vi "Format.vi"(5 "Force safe mode (false)":bool=TRUE caption="Force safe mode (true)", 7 "Restart after format (true)":bool caption="Restart after format (false)", 8 "error in (no error)":errorcluster, 10 "Network settings (reset all adapters)":T1=2 caption="Network settings (preserve all network adapters)" items=["reset primary, disable others", "preserve primary, disable others", "preserve all network adapters"], 11 "RT Management in":refnum<class "RT Management.lvclass">) -> (0 "error out":errorcluster, 3 "RT Management out":refnum<class "RT Management.lvclass">)   [LabVIEW 2016, in "RT Management.lvlib" / "RT Management.lvclass"]
doc: "Formats an RT target."
uses:
  RT Management.lvclass
  <vilib>/nisyscfg/Network Settings Format.ctl
  RT Management.lvclass/RT Management.ctl
  Get SysCfg Session.vi
  <vilib>/nisyscfg/nisyscfg.lvlib
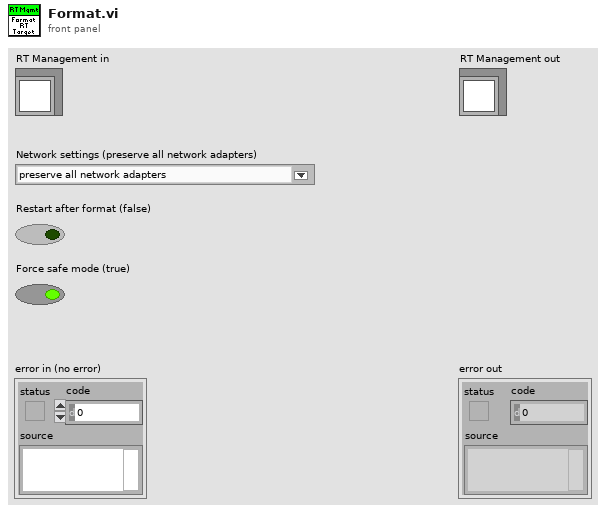
[diagram p1: front panel]
types:
  T1 = typedef "nisyscfg.lvlib/Network Settings Format.ctl" = u32
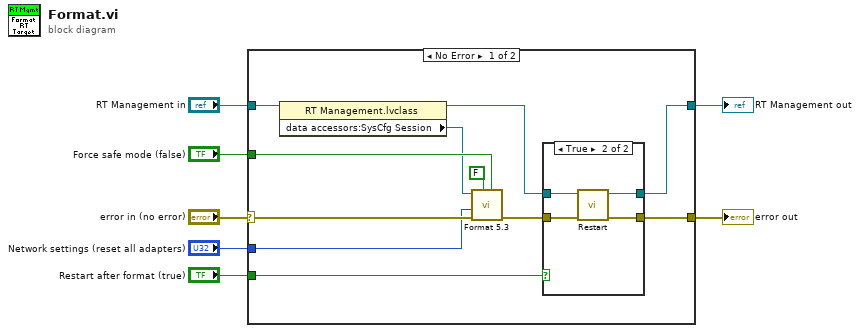
[diagram p0: block diagram]
diagram:
  n1 = case shown="No Error" "error in (no error)" {
    selector: "error in (no error)" -> [w17 w26]
    tunnel: [w11 w26] -> w6
    tunnel: [w9 w25] -> w4
    tunnel: "RT Management in" -> [w16 w25]
    tunnel: "Network settings (reset all adapters)" -> [w15 _]
    tunnel: "Restart after format (true)" -> [w10 _]
    tunnel: "Force safe mode (false)" -> [w14 _]
    frame No Error {
      n2 = property class="RT Management.lvclass"(reference=w16) -> (reference out=w18:refnum<class "RT Management.lvclass">, "data accessors:SysCfg Session"=w13:refnum<k21>)  [unwired: 1 in, 1 out]
      n3 = call <vilib>:"Format 5.3.vi"("Force Safe Mode (F)"=w14, "Restart After Format (T)"=FALSE ("restart after format (T)"), "error in (no error)"=w17, "Network Settings (reset all adapters)"=w15, "Session in"=w13) -> ("error out"=w12:errorcluster)  [unwired: 5 in, 1 out]
      n4 = case shown="True" w10 {
        tunnel: w12 -> [w20 w24]
        tunnel: [w20 w23] -> w11
        tunnel: w18 -> [w19 w22]
        tunnel: [w19 w21] -> w9
        frame False {
        }
        frame True {
          n5 = call "Restart.vi"("error in (no error)"=w24, "RT Management in"=w22) -> ("error out"=w23:errorcluster, "RT Management out"=w21:refnum<class "RT Management.lvclass">)  [unwired: 7 in]
        }
      }
    }
    frame Error {
    }
  }
  "error out" <- w6
  "RT Management out" <- w4
